vi "Get Equalization Mode.vi"(8 "error in":errorcluster, 11 "eye scan in":refnum<class "niHighSpeedSerial Eye Scan v1 Host.lvclass">) -> (0 "error out":errorcluster, 2 "equalization mode":T1, 3 "eye scan out":refnum<class "niHighSpeedSerial Eye Scan v1 Host.lvclass">)   [LabVIEW 2014, in "niHighSpeedSerial Eye Scan v1 Host.lvclass"]
doc: "Returns the Equalization Mode.\n\n<B>Input Parameters</B>\n\n<B>error in</B> describes error conditions that occur before this node runs. This input provides standard 'error in' functionality.\n\n<B>eye scan in</B> Takes in a reference to your session from the previous VI.\n\n<B>Output Parameters</B>\n\n<B>error out</B> contains error information. This output provides standard 'error out' functionality.\n\n<B>equalization mode</B> indicates the Equalization Mode that the lane is using.\nenum values: DFE,LPM\n\n<B>eye scan out</B> passes a reference to your session to the next VI."
uses:
  <instrlib>/niHighSpeedSerial/Eye Scan/v1/Host/Eye Scan/niHighSpeedSerial Eye Scan v1 Host.lvclass
  <instrlib>/niHighSpeedSerial/Eye Scan/v1/Host/Common/Public/Equalization Mode.ctl
  <instrlib>/niHighSpeedSerial/Eye Scan/v1/Host/Eye Scan/niHighSpeedSerial Eye Scan v1 Host.lvclass/niHighSpeedSerial Eye Scan v1 Host.ctl
  <vilib>/Utility/error.llb/Error Cluster From Error Code.vi
  <vilib>/ErrorRing/Error Ring.xnode
  <instrlib>/niHighSpeedSerial/Eye Scan/v1/Host/Common/niHighSpeedSerial Eye Scan Common v1 Host.lvlib
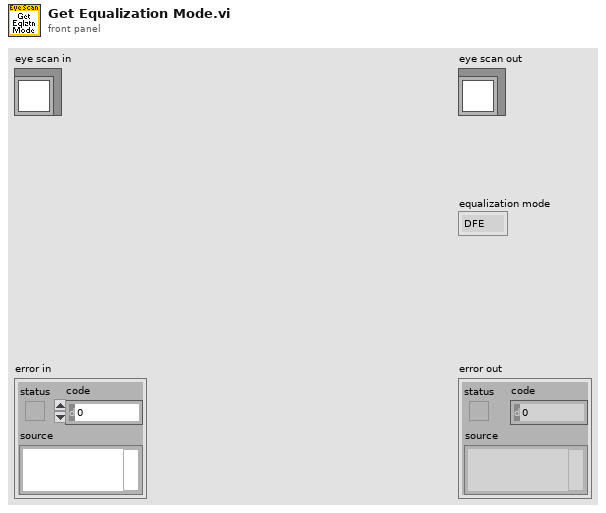
[diagram p1: front panel]
types:
  T1 = typedef "niHighSpeedSerial Eye Scan Common v1 Host.lvlib/Equalization Mode.ctl" = enum16{"DFE", "LPM"}
  T2 = typedef "niHighSpeedSerial Eye Scan v1 Host.lvclass/Private Data.ctl" = cluster{"instruction target":refnum<class "niInstr Instruction Target v1 Host.lvclass">, "channels":T3[], "measure state":T4, "rx output divider":T5, "equalization mode":T1, "rx data width":T6, "BER floor":dbl, "number of points completed":i32, "rx output divider configured?":bool, "equalization mode configured?":bool, "rx data width configured?":bool}
  T3 = typedef "niHighSpeedSerial Eye Scan v1 Host.lvclass/Channel Data.ctl" = cluster{"instance":u8, "channel":refnum<class "niHighSpeedSerial Eye Scan Single Point v1 Host.lvclass">, "point iterator":refnum<class "niHighSpeedSerial Eye Scan Point Iterator v1 Host.lvclass">}
  T4 = typedef "niHighSpeedSerial Eye Scan v1 Host.lvclass/Measure State.ctl" = enum16{"Uninitialized", "Initialized", "Ready", "Measuring", "Finished", "Aborted"}
  T5 = typedef "niHighSpeedSerial Eye Scan Common v1 Host.lvlib/RX Output Divider.ctl" = enum16{"1", "2", "4", "8", "16"}
  T6 = typedef "niHighSpeedSerial Eye Scan Common v1 Host.lvlib/Data Width.ctl" = enum16{"16 Bit", "20 Bit", "32 Bit", "40 Bit"}
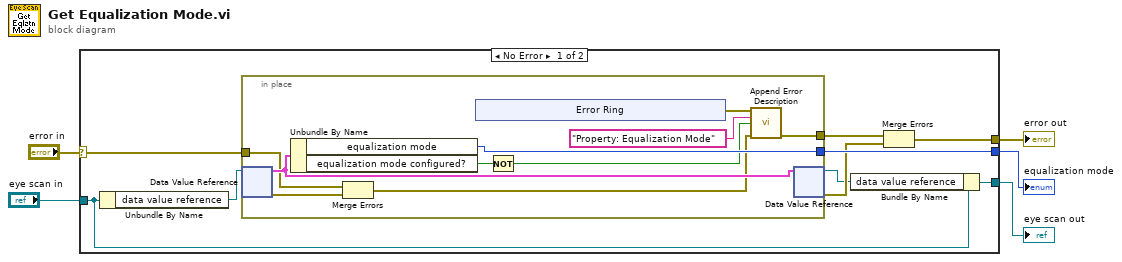
[diagram p0: block diagram]
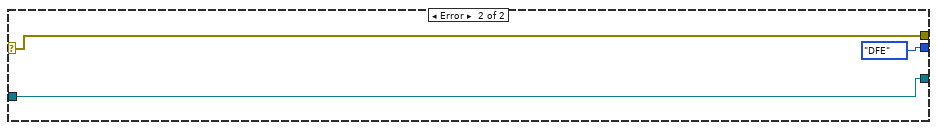
[diagram p2: hidden frame]
diagram:
  n1 = case shown="No Error" "error in" {
    selector: "error in" -> [w6 w31]
    tunnel: [w10 w31] -> w4
    tunnel: [w7 w30] -> w2
    tunnel: "eye scan in" -> [w8 w30]
    tunnel: [w13 Equalization_Mode."DFE" ("Equalization Mode")] -> w1
    frame No Error {
      n2 = Unbundle By Name(w8) -> ("data value reference"=w14:refnum<data-value>)
      n3 = in-place {
        in-place-border: [w24] -> w13
        in-place-border: [w18] -> w12
        in-place-border: w6 -> [w22]
        n4 = in-place-dvr #1(w14) -> (w23:T2, w21:errorcluster)
        n5 = Unbundle By Name(w23) -> ("equalization mode"=w24:T1, "equalization mode configured?"=w17:bool)
        n6 = Merge Errors(w22, w21) -> (w19:errorcluster)
        n7 = xnode "Error Ring"() -> ("error out"=w20:errorcluster)
        n8 = Not(x=w17) -> (.not. x?=w16:bool)
        n9 = call <instrlib>:"Append Error Description.vi"("error to append"=w20, "append string (\"\")"="Property: Equalization Mode" ("replace string (\"\")"), "generate error?"=w16, "error in"=w19) -> ("error out"=w18:errorcluster)  [unwired: 11 in]
        n10 = in-place-dvr #1(w23) -> (w9:refnum<data-value>, w11:errorcluster)
      }
      n11 = Bundle By Name(cluster=w8, "data value reference"=w9) -> (w7:refnum<class "niHighSpeedSerial Eye Scan v1 Host.lvclass">)
      n12 = Merge Errors(w12, w11) -> (w10:errorcluster)
    }
    frame Error {
    }
  }
  "error out" <- w4
  "eye scan out" <- w2
  "equalization mode" <- w1
